vi "Conv1D_CuLab.vi"(6 "Kernel Relative Size":sgl=0.001, 7 "No. of Repetition":i32, 11 "Size":i32) -> (3 "Results(s)":dbl format="%.7f")   [LabVIEW 2020]
uses:
  13ac56ee-d342-4fc9-916d-ee8b581d680f.vi
  e733ec95-1f17-4a92-a93c-f13053a3e0ea.vi
  <vilib>/Ngene/CuLab - GPU Accelerated Toolkit/Toolkit/Low_Level/Tensor_Classes/T_Children/T1D/T1D_Children/T1D_SGL/Pull.vi
  <vilib>/Utility/High Resolution Relative Seconds.vi
  <vilib>/Ngene/CuLab - GPU Accelerated Toolkit/Toolkit/Low_Level/GPU_Wrapper/cudart/Memory/PULL/1D/cudart_PULL_Data(SGL_1D).vi
  <vilib>/Ngene/CuLab - GPU Accelerated Toolkit/Toolkit/Low_Level/Tensor_Classes/T_Children/T1D/T1D_Children/T1D_SGL/T1D_SGL.lvclass
  C:/Program Files/National Instruments/LabVIEW 2020/vi.lib/Ngene/CuLab - GPU Accelerated Toolkit/Toolkit/Low_Level/Tensor_Classes/Tensor.lvclass
  C:/Program Files/National Instruments/LabVIEW 2020/vi.lib/Ngene/CuLab - GPU Accelerated Toolkit/Toolkit/Low_Level/Tensor_Classes/T_Children/T1D/T1D.lvclass
  <vilib>/Ngene/CuLab - GPU Accelerated Toolkit/Toolkit/Low_Level/Tensor_Classes/T_Children/T1D/T1D_Children/T1D_SGL/Create.vi
  <vilib>/Ngene/CuLab - GPU Accelerated Toolkit/Toolkit/Low_Level/Tensor_Classes/T_Children/T1D/T1D_Children/T1D_SGL/Push.vi
  <vilib>/Ngene/CuLab - GPU Accelerated Toolkit/Toolkit/API/Signal Processing/Signal Operation/Convolution/T1D/CU_Convolution_T1D_SGL.vi
  <vilib>/Ngene/CuLab - GPU Accelerated Toolkit/Toolkit/Low_Level/Checkers/Check_Tensor_Ref.vi
  <vilib>/Ngene/CuLab - GPU Accelerated Toolkit/Toolkit/Low_Level/Tensor_Classes/Property/Get_Mem_Desc.vi
  <vilib>/Ngene/CuLab - GPU Accelerated Toolkit/Toolkit/Low_Level/Tensor_Classes/T_Children/T1D/Property/Get_Dims.vi
  <vilib>/Ngene/CuLab - GPU Accelerated Toolkit/Toolkit/Low_Level/GPU_Wrapper/cudart/Memory/Utils/cudart_get_type_size(inBytes).vi
  <vilib>/Ngene/CuLab - GPU Accelerated Toolkit/Toolkit/Low_Level/GPU_Wrapper/cudart/cudart_get_Error_String.vi
  <vilib>/Analysis/NI_AALBase.lvlib
  <vilib>/Ngene/CuLab - GPU Accelerated Toolkit/Toolkit/CuLab.lvlib
panel:
  out "error out":errorcluster
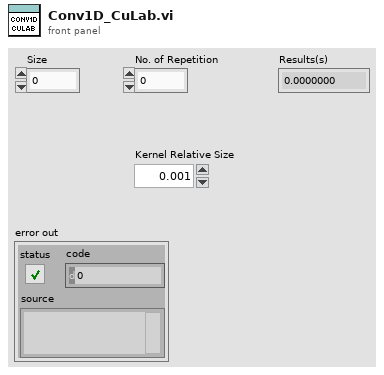
[diagram p1: front panel]
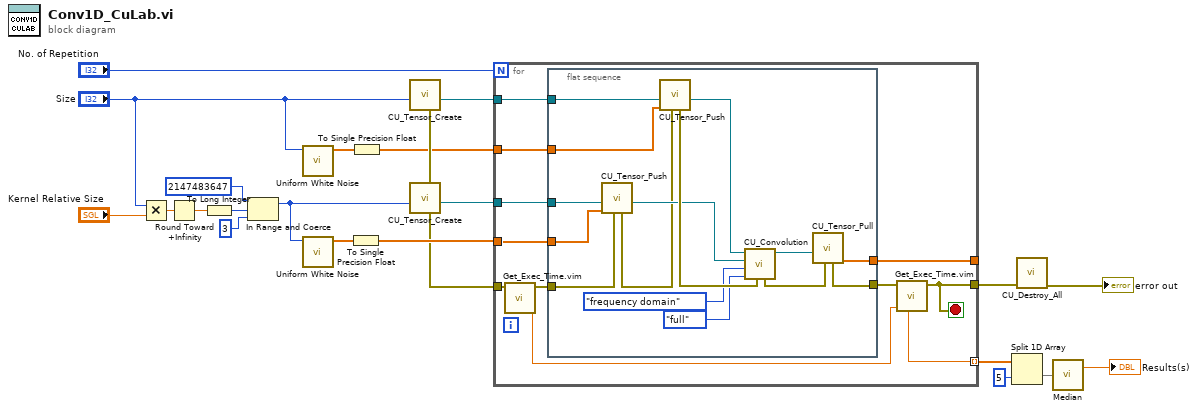
[diagram p0: block diagram]
diagram:
  n1 = Multiply(x="Size", y="Kernel Relative Size") -> (x*y=w8:sgl)
  n2 = Round Toward +Infinity(x=w8) -> (ceil(x): smallest int >= x=w7:sgl)
  n3 = To Long Integer(number=w7) -> (32bit integer=w6:i32)
  n4 = In Range and Coerce(upper limit=2147483647 ("lower limit"), x=w6, lower limit=3) -> (coerced(x)=w20:i32)  [unwired: 1 out]
  n5 = call <vilib>:"Uniform White Noise.vi"("samples"="Size") -> ("uniform white noise"=w10:dbl[])  [unwired: 9 in, 1 out]
  n6 = call <vilib>:"Uniform White Noise.vi"("samples"=w20) -> ("uniform white noise"=w11:dbl[])  [unwired: 9 in, 1 out]
  n7 = To Single Precision Float(number=w11) -> (single precision float=w16:sgl[])
  n8 = To Single Precision Float(number=w10) -> (single precision float=w12:sgl[])
  n9 = call-poly <vilib>:"CU_Tensor_Create.vi"("Length"="Size") -> ("T1D_SGL out"=w15:refnum<class "T1D_SGL.lvclass">, "error out"=w17:errorcluster)  [unwired: 9 in]
  n10 = call-poly <vilib>:"CU_Tensor_Create.vi"("error in (no error)"=w17, "Length"=w20) -> ("T1D_SGL out"=w14:refnum<class "T1D_SGL.lvclass">, "error out"=w9:errorcluster)  [unwired: 8 in]
  n11 = for {
    N: "No. of Repetition" -> [_]
    tunnel: w16 -> [w32]
    tunnel: w12 -> [w31]
    tunnel: w15 -> [w33]
    tunnel: w14 -> [w34]
    tunnel: [w25] -> w13
    tunnel: [w28] -> w18 mode=indexing
    tunnel: w9 -> [w27]
    tunnel: [w24] -> _
    stop <- w25 stop-if-true
    n12 = call "Get_Exec_Time.vim"("error in (no error)"=w27) -> ("T(n)"=w29:dbl, "error out"=w30:errorcluster)  [unwired: 6 in, 1 out]
    n13 = flat-sequence {
      tunnel: w34 -> [w48]
      tunnel: w33 -> [w47]
      tunnel: w32 -> [w43]
      tunnel: w31 -> [w42]
      tunnel: w30 -> [w41]
      tunnel: [w36] -> w26
      tunnel: [w35] -> w24
      frame #0 {
        n14 = call-poly <vilib>:"CU_Tensor_Push.vi"("error in (no error)"=w41, "CPU_Data_1D_SGL"=w43, "T1D_SGL in"=w48) -> ("T1D_SGL out"=w40:refnum<class "T1D_SGL.lvclass">, "error out"=w37:errorcluster)  [unwired: 7 in]
        n15 = call-poly <vilib>:"CU_Tensor_Push.vi"("error in (no error)"=w37, "CPU_Data_1D_SGL"=w42, "T1D_SGL in"=w47) -> ("T1D_SGL out"=w44:refnum<class "T1D_SGL.lvclass">, "error out"=w45:errorcluster)  [unwired: 7 in]
        n16 = call-poly <vilib>:"CU_Convolution.vi"("error in"=w45, "output size"=enum32{"full", "size X", "compact"}."full", "algorithm"=enum32{"direct", "frequency domain"}."frequency domain", "Y"=w40, "X"=w44) -> ("X * Y"=w46:refnum<class "T1D_SGL.lvclass">, "error out"=w49:errorcluster)  [unwired: 5 in]
        n17 = call-poly <vilib>:"CU_Tensor_Pull.vi"("error in (no error)"=w49, "T1D_SGL in"=w46) -> ("Dest out"=w35:sgl[], "error out"=w36:errorcluster)  [unwired: 7 in, 1 out]
      }
    }
    n18 = call "Get_Exec_Time.vim"("T(n-1)"=w29, "error in (no error)"=w26) -> ("error out"=w25:errorcluster, "dT"=w28:dbl)  [unwired: 5 in, 1 out]
  }
  n19 = Split 1D Array(array=w18, index=5) -> (second subarray=w3:dbl[])  [unwired: 1 out]
  n20 = call <vilib>:"CU_Destroy_All.vi"("error in"=w13) -> ("error out"=→"error out":errorcluster)  [unwired: 10 in]
  n21 = call <vilib>:"Median.vi"("X"=w3) -> ("median"=→"Results(s)":dbl)  [unwired: 1 out]
